vi "Set Table Context.vi"(8 "error in (no error)":errorcluster, 9 "Context":T1, 10 "Table Names":string[](array[string]), 11 "Stack in":T1[](array[typedef])) -> (0 "error out":errorcluster, 3 "Stack out":T1[](array[typedef]))   [LabVIEW 2017, in "TOML.lvlib"]
uses:
  TOML.lvlib
  Context.ctl
  Table Context.ctl
  Key-Value Pair.ctl
  Value.ctl
  Value Type.ctl
  Table Array Context.ctl
  <vilib>/Utility/error.llb/Error Cluster From Error Code.vi
  <vilib>/ErrorRing/Error Ring.xnode
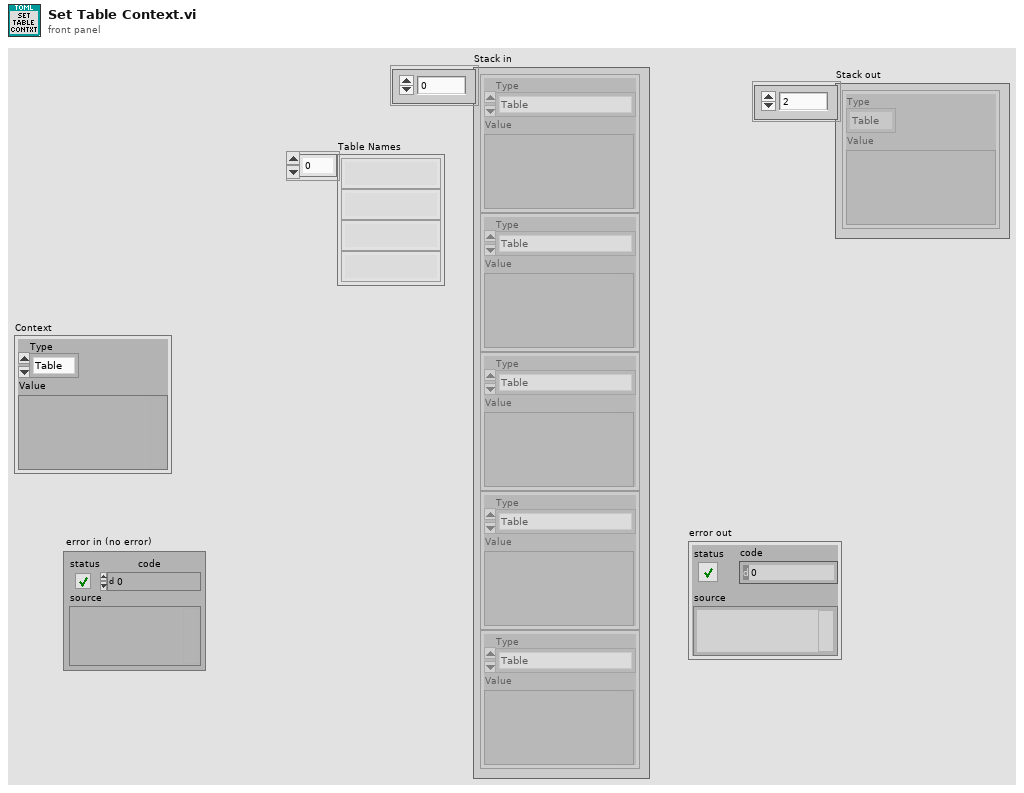
[diagram p1: front panel]
types:
  T1 = typedef "TOML.lvlib/Context.ctl" = cluster{"Type":enum16{"Table", "Array", "Inline Table", "Table Array"}, "Value":variant}
  T2 = enum16{"Table", "Array", "Inline Table", "Table Array"}
  T3 = typedef "TOML.lvlib/Value.ctl" = cluster{"Type":T4, "Value":variant}
  T4 = typedef "TOML.lvlib/Value Type.ctl" = enum16{"Table", "Array", "String", "Integer", "Float", "Boolean", "Offset Date-Time", "Local Date-Time", "Local Date", "Local Time"}
  T5 = typedef "TOML.lvlib/Table Context.ctl" = cluster{"Table":T6[], "Key":string, "Defined Keys":string[]}
  T6 = typedef "TOML.lvlib/Key-Value Pair.ctl" = cluster{"Key":string, "Value":T3}
  T7 = typedef "TOML.lvlib/Table Array Context.ctl" = cluster{"Table Array":cluster{"Table":T6[]}[], "Index":i32, "Key":string}
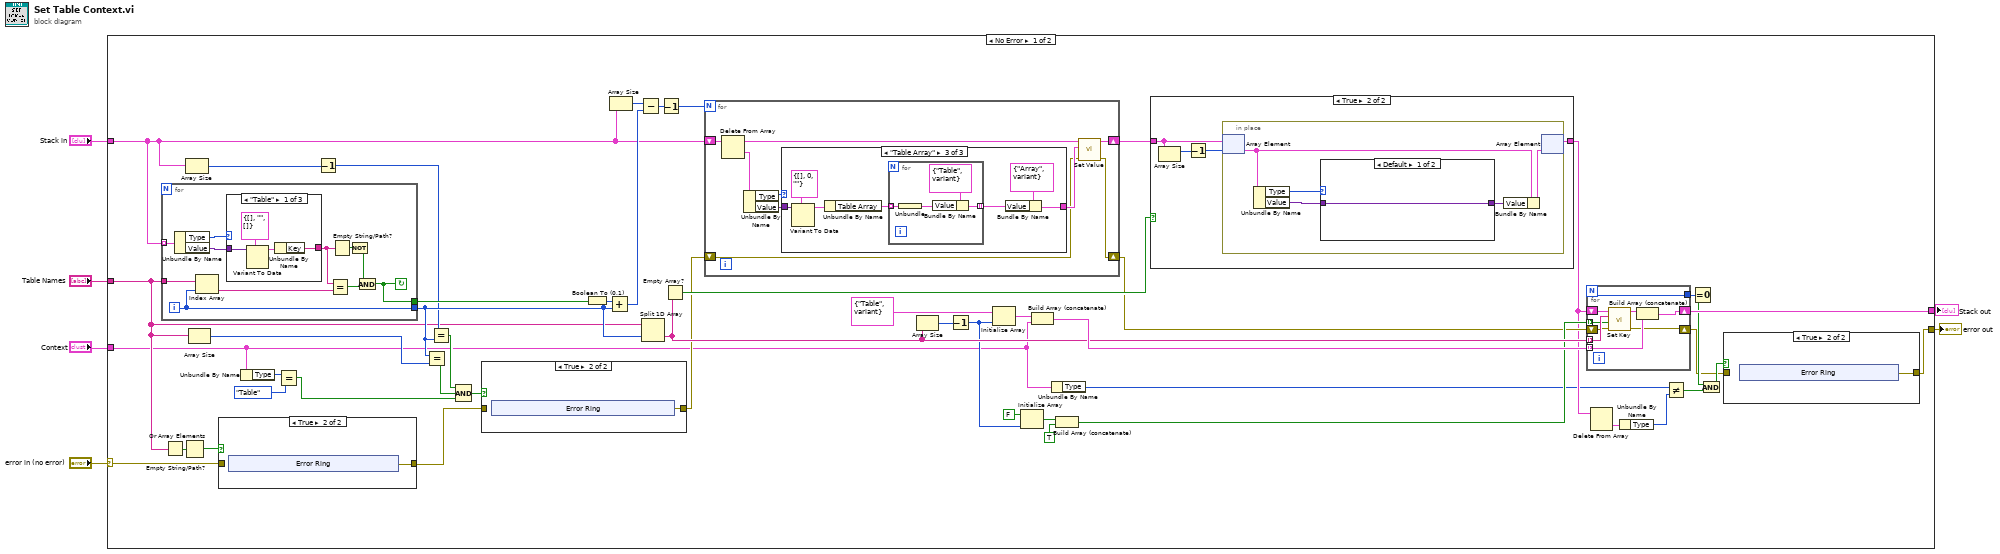
[diagram p0: block diagram]
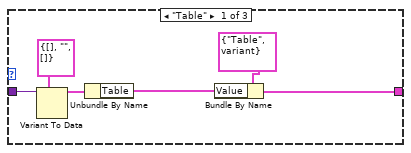
[diagram p5: hidden frame]
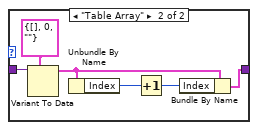
[diagram p8: hidden frame]
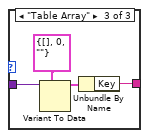
[diagram p10: hidden frame]
diagram:
  n1 = case shown="No Error" "error in (no error)" {
    selector: "error in (no error)" -> [w19 w144]
    tunnel: [w49 w145] -> w6
    tunnel: "Context" -> [w17 _]
    tunnel: [w9 w144] -> w4
    tunnel: "Table Names" -> [w22 _]
    tunnel: "Stack in" -> [w34 w145]
    frame No Error {
      n2 = for {
        tunnel: w34 -> [w134] mode=indexing
        tunnel: w22 -> [w135]
        tunnel: [w127] -> w31
        tunnel: [w126] -> w54
        i -> [w127]
        stop <- w126 continue-if-true
        n3 = Unbundle By Name(w134) -> ("Type"=w133:T2, "Value"=w132:variant)
        n4 = Index Array(array=w135, index=w127) -> (element=w131:string)
        n5 = case shown="\"Table\"" w133 {
          tunnel: w132 -> [w139 _ w143]
          tunnel: [w136 _ w140] -> w130
          frame "Table" {
            n6 = Variant To Data(type=T5 {"Table"=[], "Key"="", "Defined Keys"=[]} ("Table Context"), Variant=w139) -> (data=w137:T5)  [unwired: 1 in, 1 out]
            n7 = Unbundle By Name(w137) -> ("Key"=w136:string)
          }
          frame Default {
          }
          frame "Table Array" {
            n8 = Variant To Data(type=T7 {"Table Array"=[], "Index"=0, "Key"=""} ("Table Array Context"), Variant=w143) -> (data=w141:T7)  [unwired: 1 in, 1 out]
            n9 = Unbundle By Name(w141) -> ("Key"=w140:string)
          }
        }
        n10 = Equal?(x=w130, y=w131) -> (x = y?=w129:bool)
        n11 = Empty String/Path?(string/path=w130) -> (empty?=w128:bool)
        n12 = Not(x=w128) -> (.not. x?=w125:bool)
        n13 = And(x=w125, y=w129) -> (x .and. y?=w126:bool)
      }
      n14 = Empty String/Path?(string/path=w22) -> (empty?=w21:bool[])
      n15 = Or Array Elements(Boolean array=w21) -> (logical OR=w7:bool)
      n16 = Array Size(array=w34) -> (size(s)=w32:i32)
      n17 = Array Size(array=w22) -> (size(s)=w33:i32)
      n18 = case shown="True" w7 {
        tunnel: [w61 w62] -> w20
        tunnel: w19 -> [w61 _]
        frame False {
        }
        frame True {
          n19 = xnode "Error Ring"() -> ("error out"=w62:errorcluster)
        }
      }
      n20 = Unbundle By Name(w17) -> ("Type"=w25:T2)
      n21 = Equal?(x=w25, y=T2."Table") -> (x = y?=w23:bool)
      n22 = Decrement(x=w32) -> (x-1=w26:i32)
      n23 = Equal?(x=w31, y=w33) -> (x = y?=w29:bool)
      n24 = Equal?(x=w26, y=w31) -> (x = y?=w28:bool)
      n25 = Compound Arithmetic op=AND(w28, w29, w23) -> (w30:bool)
      n26 = case shown="True" w30 {
        tunnel: w20 -> [w67 _]
        tunnel: [w67 w68] -> w27
        frame False {
        }
        frame True {
          n27 = xnode "Error Ring"() -> ("error out"=w68:errorcluster)
        }
      }
      n28 = Boolean To (0,1)(Boolean=w54) -> (0, 1=w53:i16)
      n29 = Add(x=w53, y=w31) -> (x+y=w50:i32)
      n30 = Array Size(array=w34) -> (size(s)=w52:i32)
      n31 = Subtract(x=w52, y=w50) -> (x-y=w51:i32)
      n32 = Split 1D Array(array=w22, index=w31) -> (second subarray=w43:string[])  [unwired: 1 out]
      n33 = Decrement(x=w51) -> (x-1=w48:i32)
      n34 = Empty Array?(array=w43) -> (empty?=w41:bool)
      n35 = for {
        N: w48 -> [_]
        shift-right: [w76] -> w42
        shift-left: w34 -> [w81]
        shift-right: [w73] -> w35
        shift-left: w27 -> [w74]
        n36 = Delete From Array(array=w81) -> (deleted portion=w78:T1, array with subset deleted=w77:T1[])  [unwired: 2 in]
        n37 = Unbundle By Name(w78) -> ("Type"=w79:T2, "Value"=w80:variant)
        n38 = case shown="\"Table Array\"" w79 {
          tunnel: w80 -> [w87 _ w94]
          tunnel: [w82 _ w88] -> w75
          frame "Table" {
            n39 = Variant To Data(type=T5 {"Table"=[], "Key"="", "Defined Keys"=[]} ("Table Context"), Variant=w87) -> (data=w85:T5)  [unwired: 1 in, 1 out]
            n40 = Unbundle By Name(w85) -> ("Table"=w83:T6[])
            n41 = Bundle By Name(cluster=T3 {"Type"=enum."Table", "Value"=variant} ("Value"), "Value"=w83) -> (w82:T3)
          }
          frame Default {
          }
          frame "Table Array" {
            n42 = Variant To Data(type=T7 {"Table Array"=[], "Index"=0, "Key"=""} ("Table Array Context"), Variant=w94) -> (data=w92:T7)  [unwired: 1 in, 1 out]
            n43 = Unbundle By Name(w92) -> ("Table Array"=w91:cluster{"Table":T6[]}[])
            n44 = for {
              tunnel: w91 -> [w98] mode=indexing
              tunnel: [w95] -> w89 mode=indexing
              n45 = Unbundle(w98) -> ("Table"=w96:T6[])
              n46 = Bundle By Name(cluster=T3 {"Type"=enum."Table", "Value"=variant} ("Value"), "Value"=w96) -> (w95:T3)
            }
            n47 = Bundle By Name(cluster=T3 {"Type"=enum."Array", "Value"=variant} ("Value"), "Value"=w89) -> (w88:T3)
          }
        }
        n48 = call "Set Value.vi"("error in (no error)"=w74, "Value"=w75, "Context in"=w77) -> ("error out"=w73:errorcluster, "Context out"=w76:T1[])  [unwired: 5 in, 2 out]
      }
      n49 = Array Size(array=w43) -> (size(s)=w47:i32)
      n50 = Decrement(x=w47) -> (x-1=w40:i32)
      n51 = Initialize Array(T1 {"Type"=enum."Table", "Value"=variant} ("Context"), w40) -> (w45:T1[])
      n52 = Initialize Array(FALSE, w40) -> (w38:bool[])
      n53 = Build Array (concatenate)(w45, w17) -> (w44:T1[])
      n54 = Unbundle By Name(w17) -> ("Type"=w13:T2)
      n55 = Build Array (concatenate)(w38, TRUE) -> (w36:bool[])
      n56 = case shown="True" w41 {
        tunnel: w42 -> [w99 w103]
        tunnel: [w99 w102] -> w16
        frame False {
        }
        frame True {
          n57 = Array Size(array=w103) -> (size(s)=w101:i32)
          n58 = Decrement(x=w101) -> (x-1=w100:i32)
          n59 = in-place {
            n60 = in-place-array #1(w103, w100) -> (w106:T1)
            n61 = Unbundle By Name(w106) -> ("Type"=w108:T2, "Value"=w107:variant)
            n62 = case shown="Default" w108 {
              tunnel: w107 -> [w109 w115]
              tunnel: [w109 w110] -> w105
              frame Default {
              }
              frame "Table Array" {
                n63 = Variant To Data(type=T7 {"Table Array"=[], "Index"=0, "Key"=""} ("Table Array Context"), Variant=w115) -> (data=w113:T7)  [unwired: 1 in, 1 out]
                n64 = Unbundle By Name(w113) -> ("Index"=w111:i32)
                n65 = Increment(x=w111) -> (x+1=w112:i32)
                n66 = Bundle By Name(cluster=w113, "Index"=w112) -> (w110:T7)
              }
            }
            n67 = Bundle By Name(cluster=w106, "Value"=w105) -> (w104:T1)
            n68 = in-place-array #1(w104) -> (w102:T1[])  [unwired: 1 out]
          }
        }
      }
      n69 = for {
        N -> [w116]
        shift-right: [w122] -> w49
        shift-left: w16 -> [w124]
        tunnel: w43 -> [w123] mode=indexing
        tunnel: w44 -> [w121] mode=indexing
        tunnel: w36 -> [w119] mode=indexing
        shift-right: [w117] -> w8
        shift-left: w35 -> [w118]
        tunnel: [w116] -> w18
        n70 = call "Set Key.vi"("error in (no error)"=w118, "Define"=w119, "Key"=w123, "Stack in"=w124) -> ("error out"=w117:errorcluster, "Stack out"=w120:T1[])  [unwired: 6 in]
        n71 = Build Array (concatenate)(w120, w121) -> (w122:T1[])
      }
      n72 = Delete From Array(array=w16) -> (deleted portion=w15:T1)  [unwired: 2 in, 1 out]
      n73 = Unbundle By Name(w15) -> ("Type"=w14:T2)
      n74 = Not Equal?(x=w13, y=w14) -> (x != y?=w12:bool)
      n75 = Equal To 0?(x=w18) -> (x = 0?=w11:bool)
      n76 = And(x=w11, y=w12) -> (x .and. y?=w10:bool)
      n77 = case shown="True" w10 {
        tunnel: [w55 w56] -> w9
        tunnel: w8 -> [w55 _]
        frame False {
        }
        frame True {
          n78 = xnode "Error Ring"() -> ("error out"=w56:errorcluster)
        }
      }
    }
    frame Error {
    }
  }
  "Stack out" <- w6
  "error out" <- w4
